vi "comm_IDN_keithley.vi"() -> ()   [LabVIEW 2024]
panel:
  out "IDent":string
  in  "Nom de ressource VISA":refnum<visa-resource-name>
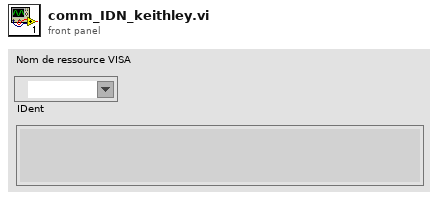
[diagram p1: front panel]
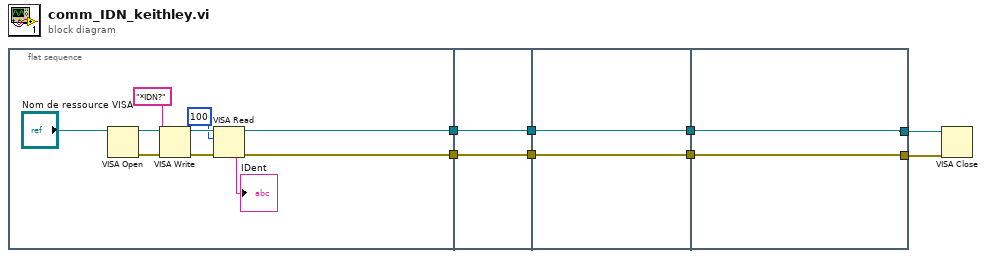
[diagram p0: block diagram]
diagram:
  n1 = flat-sequence {
    tunnel: [w11] -> w4
    tunnel: [w10] -> w1
    tunnel: [w20] -> w5
    tunnel: w4 -> [w20]
    tunnel: [w19] -> w2
    tunnel: w1 -> [w19]
    tunnel: [w22] -> w6
    tunnel: w5 -> [w22]
    tunnel: [w21] -> w3
    tunnel: w2 -> [w21]
    tunnel: [w24] -> w7
    tunnel: [w23] -> w8
    tunnel: w6 -> [w24]
    tunnel: w3 -> [w23]
    frame #0 {
      n2 = VISA Open(VISA resource name="Nom de ressource VISA") -> (VISA resource name=w17:refnum<visa-resource-name>, error out=w9:errorcluster)  [unwired: 4 in]
      n3 = VISA Write(VISA resource name=w17, write buffer="*IDN?" ("buffer d'écriture"), error in (no error)=w9) -> (VISA resource name out=w14:refnum<visa-resource-name>, error out=w15:errorcluster)  [unwired: 1 out]
      n4 = VISA Read(VISA resource name=w14, byte count=u32 100 ("nombre d'octets"), error in (no error)=w15) -> (VISA resource name out=w11:refnum<visa-resource-name>, read buffer=→"IDent":string, error out=w10:errorcluster)  [unwired: 1 out]
    }
    frame #1 {
    }
    frame #2 {
    }
    frame #3 {
    }
  }
  n5 = VISA Close(VISA resource name=w7, error in (no error)=w8) -> ()  [unwired: 1 out]
